vi "GV gated frame clock.vi"() -> ()   [LabVIEW 2017]
panel:
  out "Gated frame clock":bool
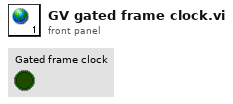
[diagram p1: front panel]
diagram:
